vi "Process one Action.vi"(8 "RPC notifier in":refnum<notifier>, 9 "Server":bool, 10 "First Byte":u8, 11 "connection ID":refnum<k5>) -> (0 "Debug Sring":string, 3 "NT Event Data":T1={"Operation"=enum."Assign", "Name"="", "Field Value"={"Dbl"=0.0, "String"="kjn", "Type"=enum."String", "Boolean"=FALSE, "Sequence #"=0, "Flags"=0}})   [LabVIEW 2017]
doc: "This VI handles one pending NT transaction. It outputs a debug string that could be helpful if a client doesn't adhere to the standard or if some other framing issues occur. The code is largely the same for client and server, so a parameter is used to identify which type is doing the processing. The RPC notifier is used to invoke functions based based on NT RPC requests."
uses:
  <vilib>/Rock Robotics/Network Tables/NT Event Type.ctl
  <vilib>/Rock Robotics/Network Tables/Protocol Operations.ctl
  <vilib>/Rock Robotics/Network Tables/Field Data.ctl
  <vilib>/Rock Robotics/Network Tables/Field Type.ctl
  <vilib>/Rock Robotics/Network Tables/Sequence.ctl
  <vilib>/Rock Robotics/Network Tables/Make Table Operation.ctl
  <vilib>/Rock Robotics/Network Tables/NT Globals.vi
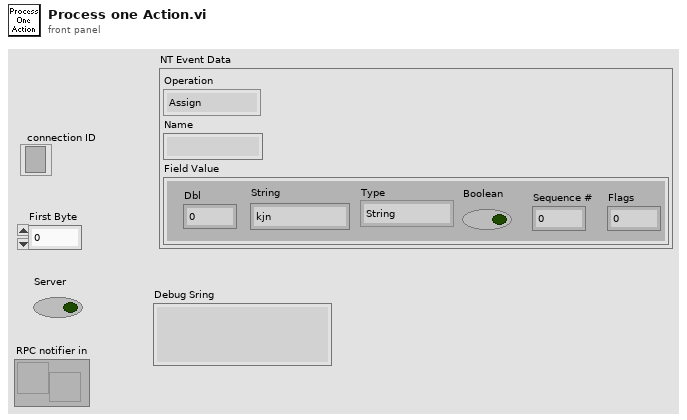
[diagram p1: front panel]
types:
  T1 = typedef "NT Event Type.ctl" = cluster{"Operation":T2, "Name":string, "Field Value":T3}
  T2 = typedef "Protocol Operations.ctl" = enum16{"Unknown", "Keep Alive", "Client Hello", "Version not supported", "Server Hello Complete", "Assign", "Update", "No Op", "Server Hello", "Client Hello Complete", "Update Flags", "Delete Entry", "Delete All", "RPC Exec", "RPC Response"}
  T3 = typedef "Field Data.ctl" = cluster{"Dbl":dbl, "String":string, "Type":T4, "Boolean":bool, "Sequence #":T5, "Flags":u8}
  T4 = typedef "Field Type.ctl" = enum8{"Invalid", "Bool", "Numeric", "String", "Raw", "Boolean Array", "Numeric Array", "String Array", "RPC"}
  T5 = typedef "Sequence.ctl" = u16
  T6 = enum16{"Add Cnx", "Remove Cnx", "Retrieve List", "Cnx Inited"}
  T7 = typedef "Make Table Operation.ctl" = enum16{"Get or Add Field", "Get Field or Add Temp", "Replace Temp ID", "Get Field ID - No Add", "Get Table Field IDs", "Get Field ID Info", "Move Field to Temp", "Validate", "Remove Field", "Remove All"}
  T8 = enum16{"Update Field", "Read Field", "Assign Field"}
  T9 = cluster{"type":u8, "ID":u16, "Seq Num":u16, "flags":u8}
  T10 = cluster{"Entry ID":u16, "Sequence #":u16, "Type":u8}
  T11 = enum16{"Add", "Remove", "Clear", "Init", "Retrieve"}
  T12 = enum16{"Update Field", "Read Field", "Assign Field", "Remove All"}
  T13 = typedef "Field ID.ctl" = i32
  T14 = cluster{"String":string, "timeout ms (25000)":u8}
  T15 = cluster{"vi reference":refnum<vi>, "TCP Network Connection out":refnum<k5>, cluster{"RPC field ID":u16, "Unique ID":u16}}
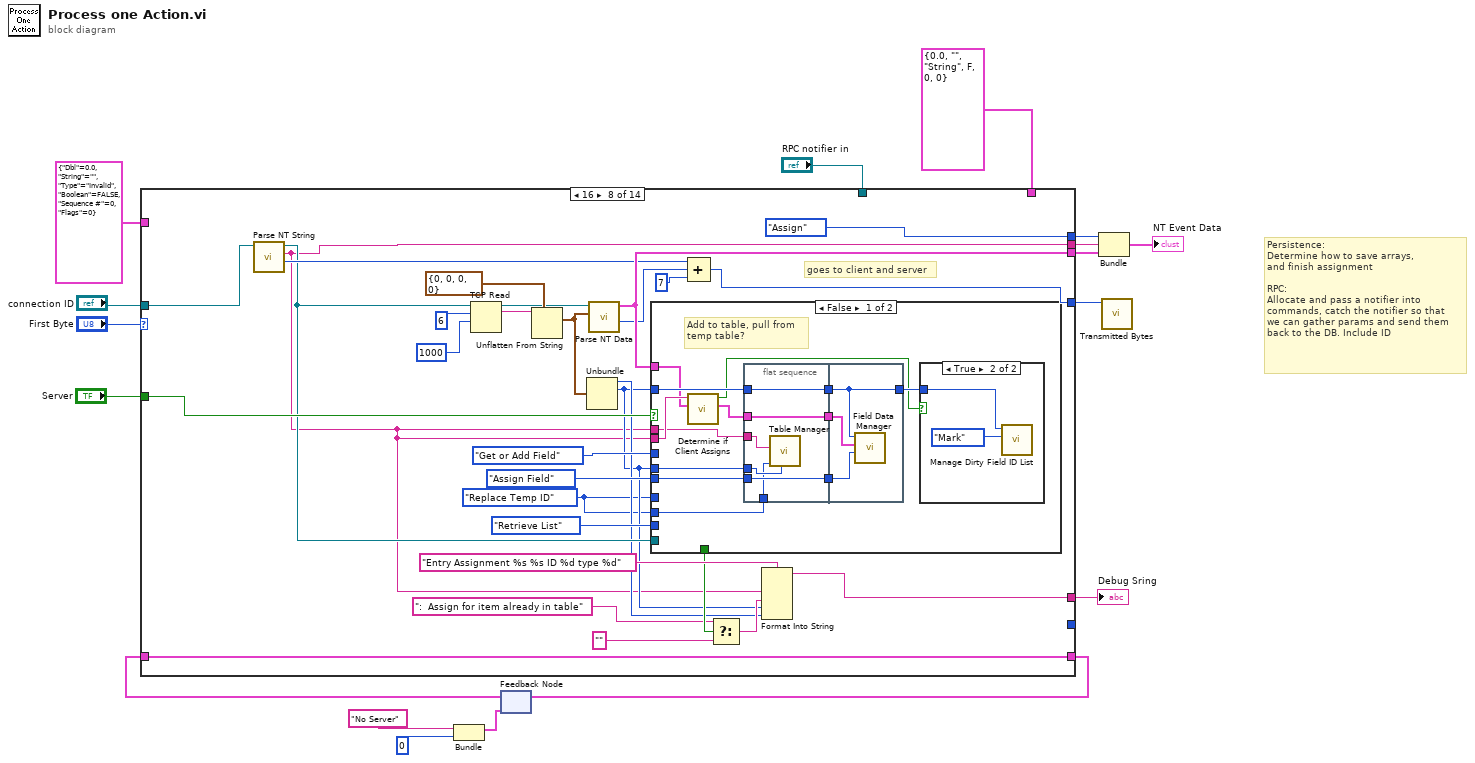
[diagram p0: block diagram]
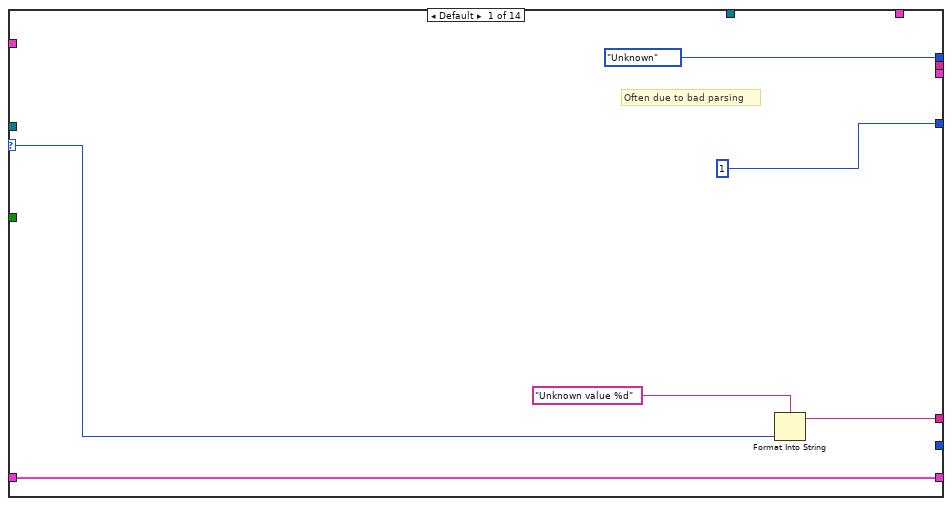
[diagram p2: hidden frame]
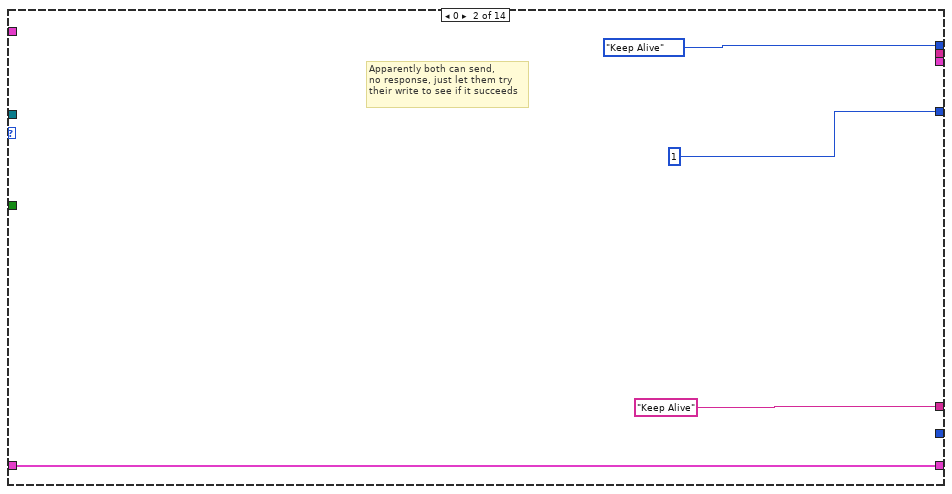
[diagram p3: hidden frame]
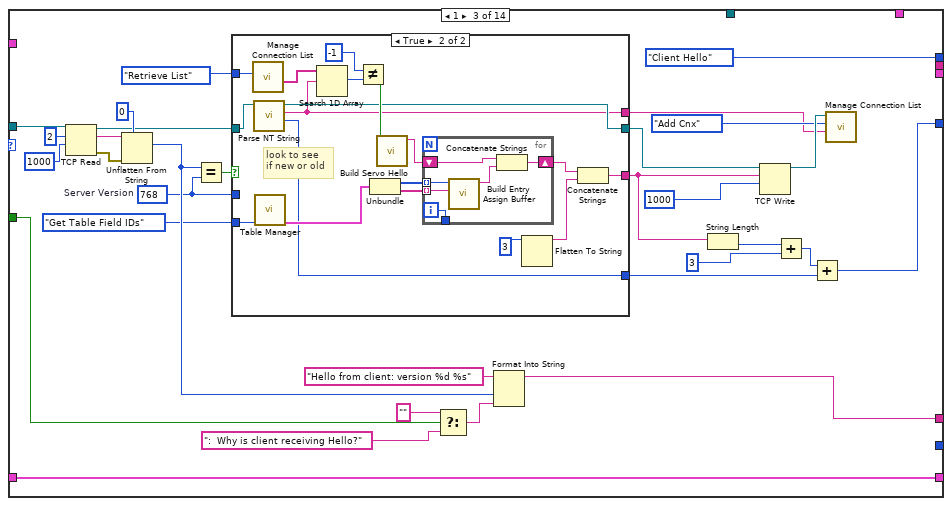
[diagram p4: hidden frame]
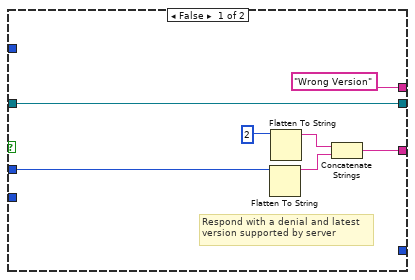
[diagram p5: hidden frame]
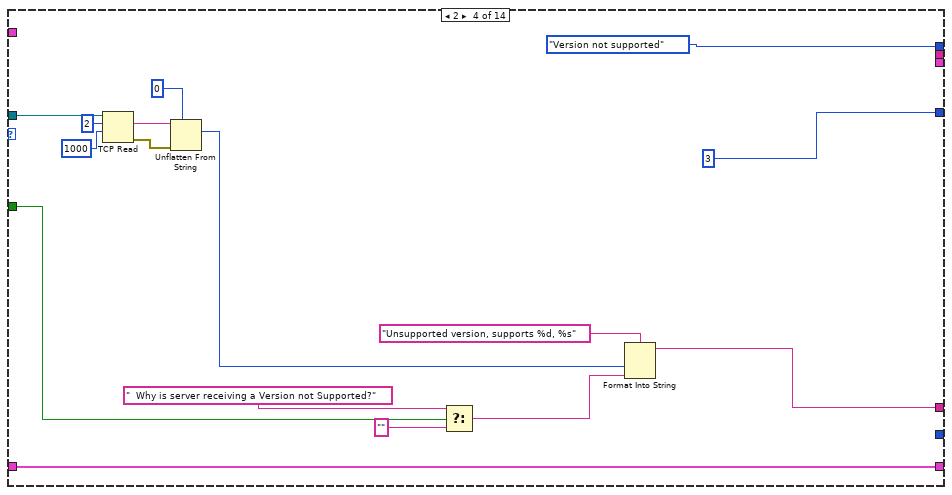
[diagram p6: hidden frame]
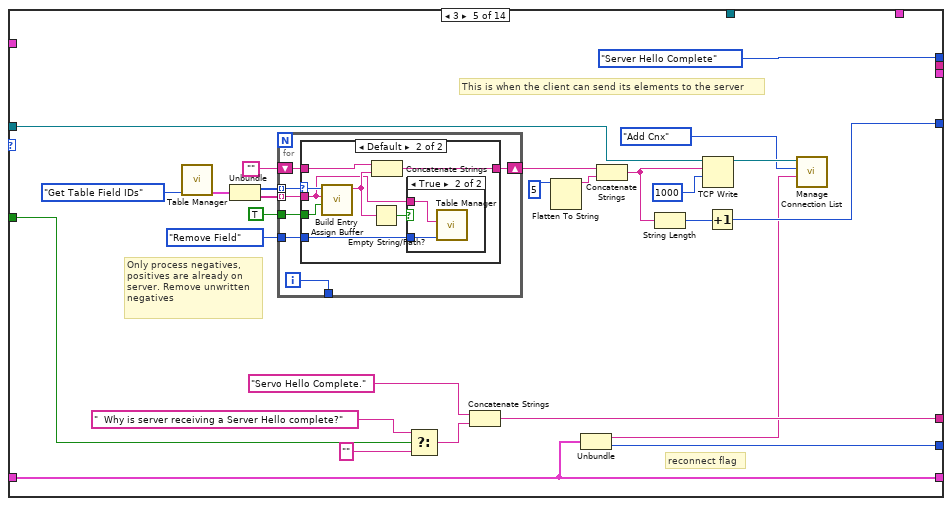
[diagram p7: hidden frame]
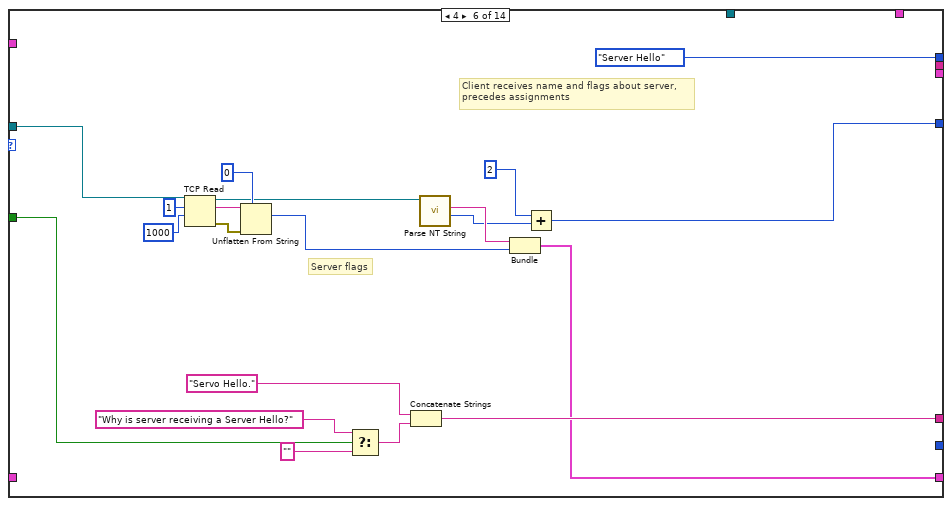
[diagram p10: hidden frame]
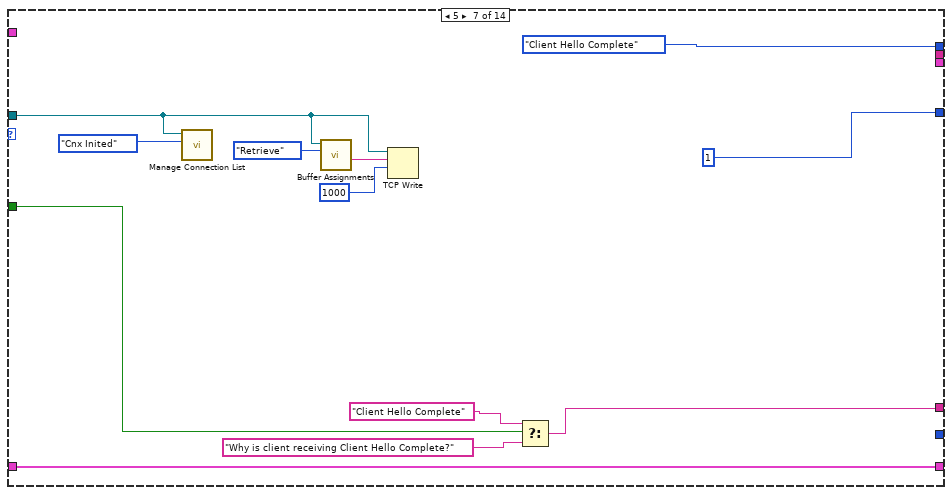
[diagram p11: hidden frame]
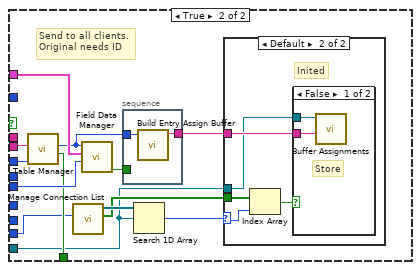
[diagram p13: hidden frame]
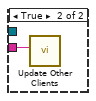
[diagram p15: hidden frame]
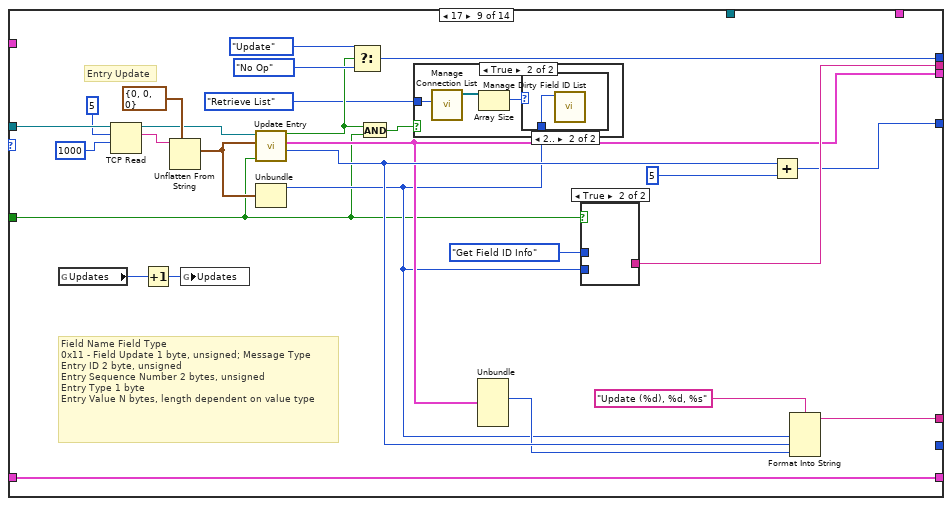
[diagram p16: hidden frame]
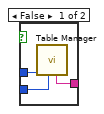
[diagram p19: hidden frame]
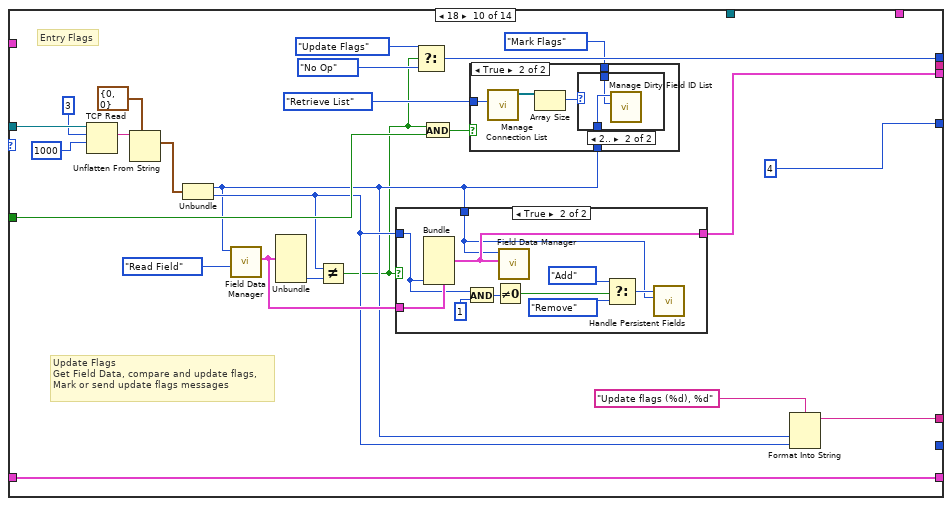
[diagram p20: hidden frame]
diagram:
  # "Persistence:\nDetermine how to save arrays,\nand finish assignment\n\nRPC:\nAllocate and pass a notifier into\ncommands, catch the notifier so that\nwe can gather params and send them\nback to the DB. Include ID"
  n1 = Bundle("No Server", "bytes to read"=u8 0) -> (w4:cluster{string, "bytes to read":u8})  [unwired: 1 in]
  n2 = feedback #1(w4) -> (w6:cluster{string, "bytes to read":u8})
  n3 = case shown="16" "First Byte" {
    selector: "First Byte" -> [w22 _ _ _ _ _ _ _ _ _ _ _ _ _]
    tunnel: "connection ID" -> [_ _ w56 w100 w129 w158 w171 w190 w283 w315 w340 w383 w439 w475]
    tunnel: "Server" -> [_ _ w43 w93 w132 w170 w178 w207 w261 w305 w348 w388 w430 w466]
    tunnel: [w21 "Keep Alive" w58 w97 w122 w164 w179 w203 w284 w316 w345 "Delete All" w433 w469] -> w14
    tunnel: [Protocol_Operations."Unknown" Protocol_Operations."Keep Alive" Protocol_Operations."Client Hello" Protocol_Operations."Version not supported" Protocol_Operations."Server Hello Complete" Protocol_Operations."Server Hello" Protocol_Operations."Client Hello Complete" Protocol_Operations."Assign" w275 w307 Protocol_Operations."Delete Entry" Protocol_Operations."Delete All" Protocol_Operations."RPC Exec" Protocol_Operations."RPC Response"] -> w12
    tunnel: [_ _ _ _ _ _ _ w183 w273 _ _ _ _ w465] -> w11
    tunnel: [_ _ _ _ _ _ _ w197 w267 w296 _ _ _ w463] -> w10
    tunnel: [1 ("timeout ms (25000)") 1 ("timeout ms (25000)") w32 3 ("timeout ms (25000)") w117 w156 1 ("timeout ms (25000)") w195 w270 4 ("timeout ms (25000)") 3 ("bytes to read") 3 ("bytes to read") w435 w471] -> w9
    tunnel: T3 {"Dbl"=0.0, "String"="", "Type"=enum."Invalid", "Boolean"=FALSE, "Sequence #"=0, "Flags"=0} ("Field Value In") -> [_ _ _ _ _ _ _ _ _ _ w337 _ _ _]
    tunnel: [w18 w24 w28 w90 w110 w154 w180 w191 w259 w294 w336 w377 w443 w478] -> w7
    tunnel: w6 -> [w18 w24 w28 w90 w110 _ w180 w191 w259 w294 w336 w377 w443 w478]
    tunnel: [_ _ _ _ w108 _ _ _ _ _ _ _ _ _] -> _
    tunnel: "RPC notifier in" -> [_ _ _ _ _ _ _ _ _ _ _ _ w413 _]
    tunnel: T3 {"Dbl"=0.0, "String"="", "Type"=enum."String", "Boolean"=FALSE, "Sequence #"=0, "Flags"=0} ("Field Value") -> [_ _ _ _ _ _ _ _ _ _ _ _ _ w464]
    frame Default {
      # "Often due to bad parsing"
      n4 = Format Into String(format string="Unknown value %d" ("message"), w22) -> (resulting string=w21:string)  [unwired: 2 in, 1 out]
    }
    frame 0 {
      # "Apparently both can send,\nno response, just let them try\ntheir write to see if it succeeds"
    }
    frame 1 {
      w48 = u16 768  # Server Version
      n5 = TCP Read(connection ID=w56, bytes to read=2, 9:1000 ("timeout ms (25000)")) -> (connection ID out=w35:refnum<k5>, data out=w53:string, error out=w51:errorcluster)  [unwired: 2 in]
      n6 = Unflatten From String(type=u16 0 ("timeout ms (25000)"), binary string=w53, error in (no error)=w51) -> (value=w50:u16)  [unwired: 2 in, 2 out]
      n7 = Equal?(x=w50, y=w48) -> (x = y?=w49:bool)
      n8 = case shown="True" w49 {
        tunnel: w48 -> [w62 _]
        tunnel: Make_Table_Operation."Get Table Field IDs" ("Operation") -> [_ w83]
        tunnel: [w61 w78] -> w38
        tunnel: w35 -> [w60 w69]
        tunnel: [w60 w68] -> w34
        tunnel: [_ w66] -> w31
        tunnel: ["Wrong Version" ("t") w67] -> w30
        tunnel: T6."Retrieve List" ("Operation") -> [_ w74]
        frame False {
          # "Respond with a denial and latest\nversion supported by server"
          n9 = Flatten To String(anything=w62) -> (data string=w64:string)  [unwired: 3 in, 2 out]
          n10 = Flatten To String(anything=u8 2) -> (data string=w63:string)  [unwired: 3 in, 2 out]
          n11 = Concatenate Strings(w63, w64) -> (w61:string)
        }
        frame True {
          # "look to see\nif new or old"
          n12 = call <vilib>:"Manage Connection List.vi"("Operation"=w74) -> ("Names"=w73:string[])  [unwired: 8 in, 2 out]
          n13 = call <vilib>:"Parse NT String.vi"("TCP Network Connection in"=w69) -> ("Size"=w66:i32, "String"=w67:string, "TCP Network Connection out"=w68:refnum<k5>)  [unwired: 8 in]
          n14 = call <vilib>:"Table Manager.vi"("Operation"=w83) -> ("Entries"=w82:cluster{"Entry IDs":T13[], "Names":string[]})  [unwired: 7 in, 3 out]
          n15 = Search 1D Array(1D array=w73, element=w67) -> (index of element=w72:i32)  [unwired: 1 in]
          n16 = Not Equal?(x=-1 ("bytes to read"), y=w72) -> (x != y?=w70:bool)
          n17 = Unbundle(w82) -> ("Entry IDs"=w77:T13[], "Names"=w76:string[])
          n18 = call <vilib>:"Build Servo Hello.vi"("Familiar"=w70) -> ("String"=w75:string)  [unwired: 10 in]
          n19 = for {
            tunnel: w77 -> [w86] mode=indexing
            shift-right: [w89] -> w79
            shift-left: w75 -> [w88]
            tunnel: w76 -> [w85] mode=indexing
            tunnel: [w84] -> _
            i -> [w84]
            n20 = call <vilib>:"Build Entry Assign Buffer.vi"("Name"=w85, "Field ID"=w86) -> ("data string"=w87:string)  [unwired: 9 in]
            n21 = Concatenate Strings(w88, w87) -> (w89:string)
          }
          n22 = Flatten To String(anything=u8 3 ("bytes to read")) -> (data string=w80:string)  [unwired: 3 in, 2 out]
          n23 = Concatenate Strings(w79, w80) -> (w78:string)
        }
      }
      n24 = Select(t="", s=w43, f=":  Why is client receiving Hello?" ("message")) -> (s? t:f=w42:string)
      n25 = Format Into String(initial string="Hello from client: version %d %s", w50, w42) -> (resulting string=w58:string)  [unwired: 2 in, 1 out]
      n26 = String Length(string=w38) -> (length=w40:i32)
      n27 = TCP Write(connection ID=w34, data in=w38, 9:1000 ("timeout ms (25000)")) -> (connection ID out=w37:refnum<k5>)  [unwired: 1 in, 2 out]
      n28 = Add(x=w40, y=3 ("bytes to read")) -> (x+y=w33:i32)
      n29 = Add(x=w33, y=w31) -> (x+y=w32:i32)
      n30 = call <vilib>:"Manage Connection List.vi"("Name"=w30, "Operation"=T6."Add Cnx", "connection ID"=w37) -> ()  [unwired: 6 in, 3 out]
    }
    frame 2 {
      n31 = TCP Read(connection ID=w100, bytes to read=2, 9:1000 ("timeout ms (25000)")) -> (data out=w103:string, error out=w101:errorcluster)  [unwired: 2 in, 1 out]
      n32 = Unflatten From String(type=u16 0 ("timeout ms (25000)"), binary string=w103, error in (no error)=w101) -> (value=w98:u16)  [unwired: 2 in, 2 out]
      n33 = Select(t="  Why is server receiving a Version not Supported?" ("message"), s=w93, f="") -> (s? t:f=w91:string)
      n34 = Format Into String(format string="Unsupported version, supports %d, %s", w98, w91) -> (resulting string=w97:string)  [unwired: 2 in, 1 out]
    }
    frame 3 {
      # "Only process negatives,\npositives are already on\nserver. Remove unwritten\nnegatives"
      # "reconnect flag"
      # "This is when the client can send its elements to the server"
      n35 = call <vilib>:"Table Manager.vi"("Operation"=Make_Table_Operation."Get Table Field IDs") -> ("Entries"=w121:cluster{"Entry IDs":T13[], "Names":string[]})  [unwired: 7 in, 3 out]
      n36 = Unbundle(w121) -> ("Entry IDs"=w120:T13[], "Names"=w119:string[])
      n37 = for {
        tunnel: w120 -> [w136] mode=indexing
        shift-right: [w139] -> w114
        shift-left: "" -> [w138]
        tunnel: w119 -> [w137] mode=indexing
        tunnel: [w135] -> _
        tunnel: TRUE -> [w134]
        tunnel: Make_Table_Operation."Remove Field" ("Operation") -> [w133]
        i -> [w135]
        n38 = case shown="Default" w136 {
          selector: w136 -> [_ w143]
          tunnel: [w140 w148] -> w139
          tunnel: w138 -> [w140 w147]
          tunnel: w137 -> [_ w141]
          tunnel: w134 -> [_ w146]
          tunnel: w133 -> [_ w142]
          frame 0.. {
          }
          frame Default {
            n39 = call <vilib>:"Build Entry Assign Buffer.vi"("Only Writers"=w146, "Name"=w141, "Field ID"=w143) -> ("data string"=w145:string)  [unwired: 8 in]
            n40 = Empty String/Path?(string/path=w145) -> (empty?=w144:bool)
            n41 = Concatenate Strings(w147, w145) -> (w148:string)
            n42 = case shown="True" w144 {
              tunnel: w142 -> [_ w150]
              tunnel: w141 -> [_ w149]
              frame False {
              }
              frame True {
                n43 = call <vilib>:"Table Manager.vi"("Operation"=w150, "Entry Name"=w149) -> ()  [unwired: 6 in, 4 out]
              }
            }
          }
        }
      }
      n44 = Select(t="  Why is server receiving a Server Hello complete?" ("message"), s=w132, f="") -> (s? t:f=w124:string)
      n45 = Concatenate Strings("Servo Hello Complete.", w124) -> (w122:string)
      n46 = Flatten To String(anything=u8 5 ("bytes to read")) -> (data string=w111:string)  [unwired: 3 in, 2 out]
      n47 = Unbundle(w110) -> (w109:string, "bytes to read"=w108:u8)
      n48 = Concatenate Strings(w114, w111) -> (w113:string)
      n49 = String Length(string=w113) -> (length=w118:i32)
      n50 = TCP Write(connection ID=w129, data in=w113, 9:1000 ("timeout ms (25000)")) -> (connection ID out=w116:refnum<k5>)  [unwired: 1 in, 2 out]
      n51 = Increment(x=w118) -> (x+1=w117:i32)
      n52 = call <vilib>:"Manage Connection List.vi"("Name"=w109, "Operation"=T6."Add Cnx", "connection ID"=w116) -> ()  [unwired: 6 in, 3 out]
    }
    frame 4 {
      # "Server flags"
      # "Client receives name and flags about server,\nprecedes assignments"
      n53 = TCP Read(connection ID=w158, bytes to read=1, 9:1000 ("timeout ms (25000)")) -> (connection ID out=w153:refnum<k5>, data out=w161:string, error out=w159:errorcluster)  [unwired: 2 in]
      n54 = Unflatten From String(type=u8 0 ("timeout ms (25000)"), binary string=w161, error in (no error)=w159) -> (value=w155:u8)  [unwired: 2 in, 2 out]
      n55 = Select(t="Why is server receiving a Server Hello?" ("message"), s=w170, f="") -> (s? t:f=w166:string)
      n56 = Concatenate Strings("Servo Hello.", w166) -> (w164:string)
      n57 = call <vilib>:"Parse NT String.vi"("TCP Network Connection in"=w153) -> ("Size"=w151:i32, "String"=w152:string)  [unwired: 8 in, 1 out]
      n58 = Bundle("String"=w152, "timeout ms (25000)"=w155) -> (w154:T14)  [unwired: 1 in]
      n59 = Add(x=u8 2 ("timeout ms (25000)"), y=w151) -> (x+y=w156:i32)
    }
    frame 5 {
      n60 = call <vilib>:"Manage Connection List.vi"("Operation"=T6."Cnx Inited", "connection ID"=w171) -> ()  [unwired: 7 in, 3 out]
      n61 = call <vilib>:"Buffer Assignments.vi"("Operation"=enum16{"Append", "Retrieve"}."Retrieve", "TCP Network Connection in"=w171) -> ("TCP Data"=w172:string)  [unwired: 9 in]
      n62 = TCP Write(connection ID=w171, data in=w172, 9:1000 ("timeout ms (25000)")) -> ()  [unwired: 1 in, 3 out]
      n63 = Select(t="Client Hello Complete", s=w178, f="Why is client receiving Client Hello Complete?") -> (s? t:f=w179:string)
    }
    frame 16 {
      w184 = Make_Table_Operation."Replace Temp ID" ("Operation")
      # "goes to client and server"
      n64 = call <vilib>:"Parse NT String.vi"("TCP Network Connection in"=w190) -> ("Size"=w189:i32, "String"=w183:string, "TCP Network Connection out"=w187:refnum<k5>)  [unwired: 8 in]
      n65 = TCP Read(connection ID=w187, bytes to read=6, 9:1000 ("timeout ms (25000)")) -> (connection ID out=w192:refnum<k5>, data out=w209:string)  [unwired: 2 in, 1 out]
      n66 = Unflatten From String(type=T9 {"type"=0, "ID"=0, "Seq Num"=0, "flags"=0}, binary string=w209) -> (value=w205:T9)  [unwired: 3 in, 2 out]
      n67 = Unbundle(w205) -> ("type"=w186:u8, "ID"=w185:u16)  [unwired: 2 out]
      n68 = call <vilib>:"Parse NT Data.vi"("Cluster"=w205, "TCP Network Connection in"=w192) -> ("Size"=w193:i32, "Field Value Out"=w197:T3)  [unwired: 8 in]
      n69 = case shown="False" w207 {
        tunnel: w197 -> [w220 w246]
        tunnel: Make_Table_Operation."Get or Add Field" ("Operation") -> [_ w248]
        tunnel: w183 -> [w221 w247]
        tunnel: T8."Assign Field" ("Operation") -> [w224 w245]
        tunnel: w185 -> [w223 _]
        tunnel: w184 -> [_ _]
        tunnel: [_ w241] -> w201
        tunnel: T6."Retrieve List" ("Operation") -> [_ w240]
        tunnel: w187 -> [_ w236]
        tunnel: w185 -> [w214 _]
        tunnel: w184 -> [w213 _]
        tunnel: w183 -> [w212 _]
        frame False {
          # "Add to table, pull from\ntemp table?"
          n70 = call <vilib>:"Determine if Client Assigns.vi"("Server Value In"=w220, "Name"=w221) -> ("Assignment Value"=w219:T3, "Update Server"=w218:bool)  [unwired: 8 in]
          n71 = flat-sequence {
            tunnel: w219 -> [w230]
            tunnel: w223 -> [w231]
            tunnel: w224 -> [w232]
            tunnel: [w232] -> w217
            tunnel: [w231] -> w216
            tunnel: [w230] -> w215
            tunnel: w214 -> [w229]
            tunnel: w213 -> [w228]
            tunnel: w212 -> [w227]
            tunnel: [w234] -> w222
            tunnel: w217 -> [w235]
            tunnel: w216 -> [w234]
            tunnel: w215 -> [w233]
            frame #0 {
              n72 = call <vilib>:"Table Manager.vi"("Entry ID in"=w229, "Operation"=w228, "Entry Name"=w227) -> ()  [unwired: 5 in, 4 out]
            }
            frame #1 {
              n73 = call <vilib>:"Field Data Manager.vi"("Operation"=w235, "Field Value In"=w233, "Field ID"=w234) -> ()  [unwired: 7 in, 2 out]
            }
          }
          n74 = case shown="True" w218 {
            tunnel: w222 -> [_ w226]
            frame False {
            }
            frame True {
              n75 = call <vilib>:"Manage Dirty Field ID List.vi"("Operation"=enum16{"Mark", "Retrieve/Clear", "Mark Flags"}."Mark", "Field ID"=w226) -> ()  [unwired: 8 in, 2 out]
            }
          }
        }
        frame True {
          # "Send to all clients.\nOriginal needs ID"
          n76 = call <vilib>:"Table Manager.vi"("Operation"=w248, "Entry Name"=w247) -> ("Success"=w241:bool, "Entry ID"=w244:T13)  [unwired: 6 in, 2 out]
          n77 = call <vilib>:"Manage Connection List.vi"("Operation"=w240) -> ("Inited"=w237:bool[], "Connections List"=w239:refnum<k5>[])  [unwired: 8 in, 1 out]
          n78 = call <vilib>:"Field Data Manager.vi"("Operation"=w245, "Field Value In"=w246, "Field ID"=w244) -> ("Equal"=w242:bool)  [unwired: 7 in, 1 out]
          n79 = stacked-sequence {
            tunnel: w244 -> [w258]
            tunnel: [w257] -> w243
            tunnel: w242 -> [_]
            frame #0 {
              n80 = call <vilib>:"Build Entry Assign Buffer.vi"("Field ID"=w258) -> ("data string"=w257:string)  [unwired: 10 in]
            }
          }
          n81 = Search 1D Array(1D array=w239, element=w236) -> (index of element=w238:i32)  [unwired: 1 in]
          n82 = case shown="Default" w238 {
            selector: w238 -> [_ w251]
            tunnel: w243 -> [_ w253]
            tunnel: w237 -> [_ w252]
            tunnel: w236 -> [_ w249]
            frame -1 {
            }
            frame Default {
              # "Inited"
              n83 = Index Array(array=w252, index=w251) -> (element=w250:bool)
              n84 = case shown="False" w250 {
                tunnel: w253 -> [w255 w256]
                tunnel: w249 -> [w254 _]
                frame False {
                  # "Store"
                  n85 = call <vilib>:"Buffer Assignments.vi"("data string"=w255, "TCP Network Connection in"=w254) -> ()  [unwired: 9 in, 1 out]
                }
                frame True {
                  n86 = call <vilib>:"Update Other Clients.vi"("data string"=w256) -> ()  [unwired: 11 in]
                }
              }
            }
          }
        }
      }
      n87 = Compound Arithmetic op=ADD(w189, w193, 7 ("bytes to read")) -> (w195:i32)
      n88 = Select(t=":  Assign for item already in table" ("message"), s=w201, f="" ("message")) -> (s? t:f=w199:string)
      n89 = Format Into String(format string="Entry Assignment %s %s ID %d type %d", w183, w199, w185, w186) -> (resulting string=w203:string)  [unwired: 2 in, 1 out]
    }
    frame 17 {
      # "Field Name\tField Type\n0x11 - Field Update\t1 byte, unsigned; Message Type\nEntry ID\t2 byte, unsigned\nEntry Sequence Number\t2 bytes, unsigned\nEntry Type 1 byte\nEntry Value\tN bytes, length dependent on value type"
      # "Entry Update"
      n90 = global read "NT Globals.vi" "Updates"() -> (w272:i32)
      n91 = TCP Read(connection ID=w283, bytes to read=5 ("timeout ms (25000)"), 9:1000 ("timeout ms (25000)")) -> (connection ID out=w264:refnum<k5>, data out=w280:string)  [unwired: 2 in, 1 out]
      n92 = Increment(x=w272) -> (x+1=w271:i32)
      n93 = Unflatten From String(type=T10 {"Entry ID"=0, "Sequence #"=0, "Type"=0}, binary string=w280) -> (value=w278:T10)  [unwired: 3 in, 2 out]
      n94 = global write "NT Globals.vi" "Updates"(w271) -> ()
      n95 = call <vilib>:"Update Entry.vi"("Server"=w261, "Cluster"=w278, "TCP Network Connection in"=w264) -> ("Size"=w268:i32, "Field Value Out"=w267:T3, "Updated"=w265:bool)  [unwired: 6 in]
      n96 = Unbundle(w278) -> ("Entry ID"=w262:u16)  [unwired: 2 out]
      n97 = Select(t=Protocol_Operations."Update", s=w265, f=Protocol_Operations."No Op") -> (s? t:f=w275:T2)
      n98 = And(x=w265, y=w261) -> (x .and. y?=w263:bool)
      n99 = case shown="True" w263 {
        tunnel: T6."Retrieve List" ("Operation") -> [_ w288]
        tunnel: w262 -> [_ w287]
        frame False {
        }
        frame True {
          n100 = call <vilib>:"Manage Connection List.vi"("Operation"=w288) -> ("Connections List"=w289:refnum<k5>[])  [unwired: 8 in, 2 out]
          n101 = Array Size(array=w289) -> (size(s)=w286:i32)
          n102 = case shown="2.." w286 {
            tunnel: w287 -> [_ w290]
            frame Default {
            }
            frame 2.. {
              n103 = call <vilib>:"Manage Dirty Field ID List.vi"("Field ID"=w290) -> ()  [unwired: 9 in, 2 out]
            }
          }
        }
      }
      n104 = Unbundle(w267) -> ("Type"=w266:T4)  [unwired: 5 out]
      n105 = case shown="True" w261 {
        tunnel: w262 -> [w293 _]
        tunnel: Make_Table_Operation."Get Field ID Info" ("Operation") -> [w292 _]
        tunnel: [w291 _] -> w273
        frame False {
          n106 = call <vilib>:"Table Manager.vi"("Entry ID in"=w293, "Operation"=w292) -> ("Entry Name"=w291:string)  [unwired: 6 in, 3 out]
        }
        frame True {
        }
      }
      n107 = Add(x=w268, y=5 ("timeout ms (25000)")) -> (x+y=w270:i32)
      n108 = Format Into String(format string="Update (%d), %d, %s", w262, w268, w266) -> (resulting string=w284:string)  [unwired: 2 in, 1 out]
    }
    frame 18 {
      # "Update Flags\nGet Field Data, compare and update flags,\nMark or send update flags messages"
      # "Entry Flags"
      n109 = TCP Read(connection ID=w315, bytes to read=3 ("timeout ms (25000)"), 9:1000 ("timeout ms (25000)")) -> (data out=w312:string)  [unwired: 2 in, 2 out]
      n110 = Unflatten From String(type=cluster{"Entry ID":u16, "Flags":u8} {"Entry ID"=0, "Flags"=0}, binary string=w312) -> (value=w310:cluster{"Entry ID":u16, "Flags":u8})  [unwired: 3 in, 2 out]
      n111 = Unbundle(w310) -> ("Entry ID"=w298:u16, "Flags"=w299:u8)
      n112 = call <vilib>:"Field Data Manager.vi"("Operation"=enum16{"Update Field", "Read Field"}."Read Field", "Field ID"=w298) -> ("Field Value Out"=w300:T3)  [unwired: 8 in, 1 out]
      n113 = Unbundle(w300) -> ("Flags"=w302:u8)  [unwired: 5 out]
      n114 = Not Equal?(x=w299, y=w302) -> (x != y?=w297:bool)
      n115 = case shown="True" w297 {
        tunnel: w300 -> [w318 w328]
        tunnel: w299 -> [_ w322]
        tunnel: w298 -> [_ w319]
        tunnel: [w318 w327] -> w296
        frame False {
        }
        frame True {
          n116 = Bundle(cluster=w328, "Flags"=w322) -> (w327:T3)  [unwired: 5 in]
          n117 = And(x=w322, y=1 ("timeout ms (25000)")) -> (x .and. y?=w321:i32)
          n118 = Not Equal To 0?(x=w321) -> (x != 0?=w320:bool)
          n119 = call <vilib>:"Field Data Manager.vi"("Field Value In"=w327, "Field ID"=w319) -> ()  [unwired: 8 in, 2 out]
          n120 = Select(t=T11."Add" ("Operation"), s=w320, f=T11."Remove" ("Operation")) -> (s? t:f=w324:T11)
          n121 = call <vilib>:"Handle Persistent Fields.vi"("Field ID"=w319, "Operation"=w324) -> ()  [unwired: 9 in, 1 out]
        }
      }
      n122 = Select(t=Protocol_Operations."Update Flags", s=w297, f=Protocol_Operations."No Op") -> (s? t:f=w307:T2)
      n123 = And(x=w297, y=w305) -> (x .and. y?=w306:bool)
      n124 = case shown="True" w306 {
        tunnel: T6."Retrieve List" ("Operation") -> [_ w332]
        tunnel: w298 -> [_ w331]
        tunnel: enum16{"Mark", "Retrieve/Clear", "Mark Flags"}."Mark Flags" ("Operation") -> [_ w329]
        frame False {
        }
        frame True {
          n125 = call <vilib>:"Manage Connection List.vi"("Operation"=w332) -> ("Connections List"=w333:refnum<k5>[])  [unwired: 8 in, 2 out]
          n126 = Array Size(array=w333) -> (size(s)=w330:i32)
          n127 = case shown="2.." w330 {
            tunnel: w331 -> [_ w335]
            tunnel: w329 -> [_ w334]
            frame Default {
            }
            frame 2.. {
              n128 = call <vilib>:"Manage Dirty Field ID List.vi"("Operation"=w334, "Field ID"=w335) -> ()  [unwired: 8 in, 2 out]
            }
          }
        }
      }
      n129 = Format Into String(format string="Update flags (%d), %d", w298, w299) -> (resulting string=w316:string)  [unwired: 2 in, 1 out]
    }
    frame 19 {
      # "remove from my table,\nif server, send to other clients"
      n130 = TCP Read(connection ID=w340, bytes to read=2, 9:1000 ("timeout ms (25000)")) -> (data out=w338:string)  [unwired: 2 in, 2 out]
      n131 = Unflatten From String(type=u16 0 ("ID"), binary string=w338) -> (value=w339:u16)  [unwired: 3 in, 2 out]
      n132 = case shown="True" w348 {
        tunnel: T8."Update Field" ("Operation") -> [w355 w366]
        tunnel: Make_Table_Operation."Remove Field" ("Operation") -> [w356 w365]
        tunnel: w339 -> [w354 w364]
        tunnel: w338 -> [_ w361]
        tunnel: w337 -> [w351 w360]
        frame False {
          # "remove from table"
          n133 = call <vilib>:"Table Manager.vi"("Entry ID in"=w354, "Operation"=w356) -> ("Success"=w352:bool, "Entry ID"=w353:T13)  [unwired: 6 in, 2 out]
          n134 = case shown="True" w352 {
            tunnel: w351 -> [_ w359]
            tunnel: w355 -> [_ w358]
            tunnel: w353 -> [_ w357]
            frame False {
            }
            frame True {
              n135 = call <vilib>:"Field Data Manager.vi"("Operation"=w358, "Field Value In"=w359, "Field ID"=w357) -> ()  [unwired: 7 in, 2 out]
            }
          }
        }
        frame True {
          # "Send to all clients.\nOriginal needs ID"
          n136 = call <vilib>:"Table Manager.vi"("Entry ID in"=w364, "Operation"=w365) -> ("Success"=w362:bool, "Entry ID"=w363:T13)  [unwired: 6 in, 2 out]
          n137 = case shown="True" w362 {
            tunnel: w366 -> [_ w372]
            tunnel: w360 -> [_ w370]
            tunnel: w363 -> [_ w369]
            tunnel: w361 -> [_ w367]
            frame False {
            }
            frame True {
              n138 = call <vilib>:"Field Data Manager.vi"("Operation"=w372, "Field Value In"=w370, "Field ID"=w369) -> ("Equal"=w368:bool)  [unwired: 7 in, 1 out]
              n139 = stacked-sequence {
                tunnel: [w375] -> w371
                tunnel: w368 -> [_]
                tunnel: w367 -> [w373]
                frame #0 {
                  n140 = Flatten To String(anything=u8 19 ("bytes to read")) -> (data string=w374:string)  [unwired: 3 in, 2 out]
                  n141 = Concatenate Strings(w374, w373) -> (w375:string)
                }
              }
              n142 = call <vilib>:"Update Other Clients.vi"("data string"=w371) -> ()  [unwired: 11 in]
            }
          }
        }
      }
      n143 = Format Into String(format string="Delete Entry %d", w339) -> (resulting string=w345:string)  [unwired: 2 in, 1 out]
    }
    frame 20 {
      # "remove all from my table,\nif server, send to other clients\nNot finished"
      n144 = TCP Read(connection ID=w383, bytes to read=4, 9:1000 ("timeout ms (25000)")) -> (data out=w378:string)  [unwired: 2 in, 2 out]
      n145 = Unflatten From String(type=u32 0 ("ID"), binary string=w378) -> (value=w381:u32)  [unwired: 3 in, 2 out]
      n146 = Equal?(x=w381, y=u32 3496784506 ("ID")) -> (x = y?=w379:bool)
      n147 = case shown="True" w379 {
        tunnel: w388 -> [_ w393]
        tunnel: Make_Table_Operation."Remove All" ("Operation") -> [_ w392]
        tunnel: w378 -> [_ w391]
        frame False {
          # "Ignore it if the magig isn't there"
        }
        frame True {
          n148 = case shown="True" w393 {
            tunnel: w392 -> [w398 w400]
            tunnel: [w397 _] -> _
            tunnel: w391 -> [_ w402]
            frame False {
              # "remove from table"
              n149 = call <vilib>:"Table Manager.vi"("Entry ID in"=u32 0 ("ID"), "Operation"=w398) -> ("Success"=w397:bool, "Entry ID"=w394:T13)  [unwired: 6 in, 2 out]
              n150 = call <vilib>:"Field Data Manager.vi"("Operation"=T12."Remove All", "Field ID"=w394) -> ()  [unwired: 8 in, 2 out]
            }
            frame True {
              # "Send to all clients.\nOriginal needs ID"
              n151 = call <vilib>:"Table Manager.vi"("Entry ID in"=u32 0 ("ID"), "Operation"=w400) -> ("Entry ID"=w405:T13)  [unwired: 6 in, 3 out]
              n152 = call <vilib>:"Field Data Manager.vi"("Operation"=T12."Remove All", "Field ID"=w405) -> ("Equal"=w403:bool)  [unwired: 8 in, 1 out]
              n153 = stacked-sequence {
                tunnel: [w407] -> w404
                tunnel: w403 -> [_]
                tunnel: w402 -> [w406]
                frame #0 {
                  n154 = Flatten To String(anything=u8 20 ("bytes to read")) -> (data string=w408:string)  [unwired: 3 in, 2 out]
                  n155 = Concatenate Strings(w408, w406) -> (w407:string)
                }
              }
              n156 = call <vilib>:"Update Other Clients.vi"("data string"=w404) -> ()  [unwired: 11 in]
            }
          }
        }
      }
    }
    frame 32 {
      # "params"
      # "vers"
      # "Parse the encoded params and definition"
      # "Encoded Params Buffer"
      n157 = TCP Read(connection ID=w439, bytes to read=4, 9:1000 ("timeout ms (25000)")) -> (connection ID out=w438:refnum<k5>, data out=w440:string)  [unwired: 2 in, 1 out]
      n158 = Unflatten From String(type=cluster{"RPC field ID":u16, "Unique ID":u16} {"RPC field ID"=0, "Unique ID"=0}, binary string=w440) -> (value=w412:cluster{"RPC field ID":u16, "Unique ID":u16})  [unwired: 3 in, 2 out]
      n159 = call <vilib>:"Parse NT String.vi"("TCP Network Connection in"=w438) -> ("Size"=w437:i32, "String"=w419:string, "TCP Network Connection out"=w410:refnum<k5>)  [unwired: 8 in]
      n160 = Unbundle(w412) -> ("RPC field ID"=w428:u16)  [unwired: 1 out]
      n161 = Add(x=5 ("bytes to read"), y=w437) -> (x+y=w435:i32)
      n162 = call <vilib>:"Field Data Manager.vi"("Operation"=enum16{"Update Field", "Read Field"}."Read Field", "Field ID"=w428) -> ("Field Value Out"=w421:T3)  [unwired: 8 in, 1 out]
      n163 = Unbundle(w421) -> ("String"=w420:string)  [unwired: 5 out]
      n164 = Unflatten From String(type=u8 0 ("bytes to read"), binary string=w420) -> (rest of the binary string=w426:string)  [unwired: 3 in, 2 out]
      n165 = call <vilib>:"Convert NT String to LV String.vi"("Buffer in"=w426) -> ("String Contents"=w417:string, "Remaining String"=w424:string)  [unwired: 8 in, 1 out]
      n166 = Unflatten From String(type=u8 0 ("bytes to read"), binary string=w424) -> (rest of the binary string=w422:string, value=w423:u8)  [unwired: 3 in, 1 out]
      n167 = Open VI Reference(vi path=w417, options=8) -> (vi reference=w416:refnum<vi>)  [unwired: 4 in, 1 out]
      n168 = for {
        N: w423 -> [_]
        shift-right: [w458] -> _
        shift-left: w422 -> [w460]
        tunnel: [w457] -> w414
        shift-right: [w454] -> _
        shift-left: w419 -> [w456]
        tunnel: w416 -> [w452]
        tunnel: [w452] -> w415
        stop <- w457 stop-if-true
        # "update ctl"
        # "skip defaults"
        n169 = Unflatten From String(type=u8 0 ("bytes to read"), binary string=w460) -> (rest of the binary string=w459:string, value=w455:u8)  [unwired: 3 in, 1 out]
        n170 = call <vilib>:"Convert NT String to LV String.vi"("Buffer in"=w459) -> ("String Contents"=w451:string, "Remaining String"=w453:string)  [unwired: 8 in, 1 out]
        n171 = call <vilib>:"Consume RPC Param Data.vi"("type"=w455, "RPC String in"=w453) -> ("string out"=w458:string, "Issue"=w457:bool)  [unwired: 6 in, 2 out]
        n172 = call <vilib>:"Consume RPC Param Data.vi"("Param Name"=w451, "VI in"=w452, "type"=w455, "RPC String in"=w456) -> ("string out"=w454:string)  [unwired: 4 in, 3 out]
      }
      n173 = Select(t="RPC Execute", s=w430, f="Client received RPC execute") -> (s? t:f=w433:string)
      n174 = case shown="False" w414 {
        tunnel: w415 -> [w445 w450]
        tunnel: w413 -> [w448 _]
        tunnel: w412 -> [w447 _]
        tunnel: w410 -> [w444 _]
        frame False {
          n175 = Bundle("vi reference"=w445, "TCP Network Connection out"=w444, w447) -> (w446:T15)  [unwired: 1 in]
          n176 = Send Notification(notification=w446, notifier=w448) -> ()  [unwired: 1 in, 2 out]
        }
        frame True {
          n177 = Close Reference(reference=w450, error in (no error)=errorcluster {"status"=TRUE, "code"=-44000, "source"="RPC param issue"} ("error out")) -> ()  [unwired: 1 out]
        }
      }
    }
    frame 33 {
      # "Encoded Response Buffer"
      n178 = TCP Read(connection ID=w475, bytes to read=4, 9:1000 ("timeout ms (25000)")) -> (connection ID out=w474:refnum<k5>, data out=w465:string)  [unwired: 2 in, 1 out]
      n179 = call <vilib>:"Parse NT String.vi"("TCP Network Connection in"=w474) -> ("Size"=w473:i32, "String"=w462:string)  [unwired: 8 in, 1 out]
      n180 = Add(x=5 ("bytes to read"), y=w473) -> (x+y=w471:i32)
      n181 = Select(t="Server received RPC response", s=w466, f="RPC response") -> (s? t:f=w469:string)
      n182 = Bundle(cluster=w464, "String"=w462) -> (w463:T3)  [unwired: 5 in]
    }
  }
  "Debug Sring" <- w14
  n183 = feedback-in #1(w7) -> ()
  n184 = Bundle(w12, "data out"=w11, "Field Value"=w10) -> (→"NT Event Data":cluster{T2, "data out":string, "Field Value":T3})  [unwired: 1 in]
  n185 = call <vilib>:"Transmitted Bytes.vi"("Additional"=w9) -> ()  [unwired: 10 in, 1 out]
